vi "Get and Set Test.vi"() -> ()   [LabVIEW 2017]
uses:
  String Subset.vi
  Parsing/Parse Full Path or Item Name.vi
  Offset/Find Item Locations by Path.vi
  JSONtext.lvlib
  <vilib>/addons/_JKI Toolkits/Caraya/classes/Test/Test.lvclass
  <vilib>/addons/_JKI Toolkits/Caraya/classes/Assert/Assert.lvclass
panel:
  out "Array 2":string[](array[string])
  out "Passed":bool[](array[boolean])
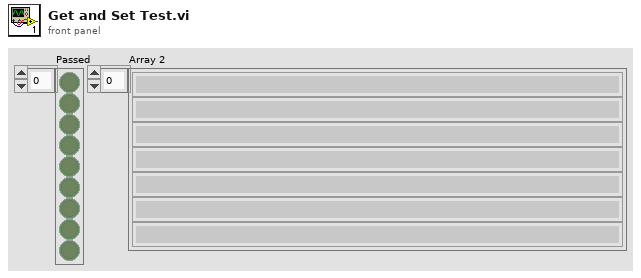
[diagram p1: front panel]
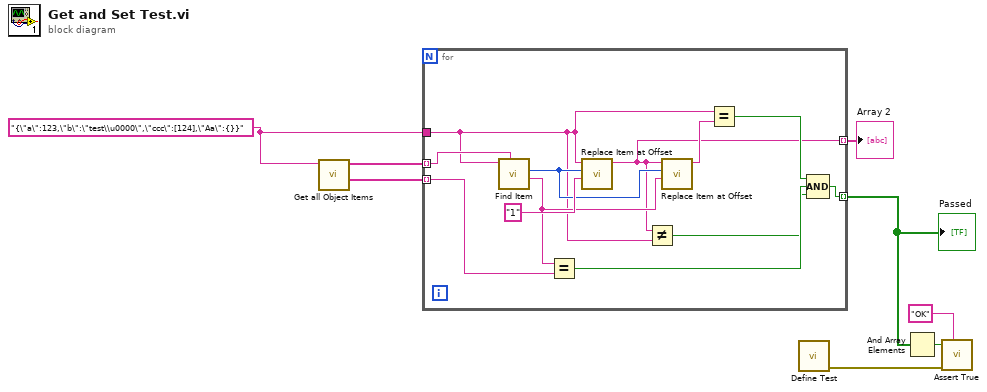
[diagram p0: block diagram]
diagram:
  w6 = "{\"a\":123,\"b\":\"test\\u0000\",\"ccc\":[124],\"Aa\":{}}"
  n1 = call "Get all Object Items.vi"("JSON"=w6) -> ("<JSON>"=w8:string[], "Item Names"=w7:string[])  [unwired: 7 in, 2 out]
  n2 = for {
    tunnel: w6 -> [w11]
    tunnel: w8 -> [w19] mode=indexing
    tunnel: w7 -> [w20] mode=indexing
    tunnel: [w16] -> w1 mode=indexing
    tunnel: [w9] -> w5 mode=indexing
    n3 = call "Find Item.vi"("$Path or Item Name"=w20, "JSON"=w11) -> ("<JSON>"=w14:string, "Item offset"=w13:i32)  [unwired: 6 in, 2 out]
    n4 = Equal?(x=w14, y=w19) -> (x = y?=w18:bool)
    n5 = call "Replace Item at Offset.vi"("New JSON Item"="1" ("JSON to Insert"), "Offset of Item to Replace"=w13, "JSON"=w11) -> ("<JSON>"=w9:string)  [unwired: 7 in, 1 out]
    n6 = Not Equal?(x=w9, y=w11) -> (x != y?=w10:bool)
    n7 = call "Replace Item at Offset.vi"("New JSON Item"=w14, "Offset of Item to Replace"=w13, "JSON"=w9) -> ("<JSON>"=w12:string)  [unwired: 7 in, 1 out]
    n8 = Equal?(x=w11, y=w12) -> (x = y?=w17:bool)
    n9 = Compound Arithmetic op=AND(w17, w18, w10) -> (w16:bool)
  }
  "Passed" <- w1
  "Array 2" <- w5
  n10 = call <vilib>:"Define Test.vi"() -> ("error out"=w2:errorcluster)  [unwired: 11 in]
  n11 = And Array Elements(Boolean array=w1) -> (logical AND=w4:bool)
  n12 = call <vilib>:"Assert True.vi"("Label"="OK", "error in (no error)"=w2, "True?"=w4) -> ()  [unwired: 8 in, 1 out]
